vi "niScope Signalize Abort to Digitizing Process.vi"(8 "error in":errorcluster, 10 "send abort signal? (True)":bool=TRUE, 11 "niScope in":T1={"channel cfg"=[], "sessions"=[], "multi cards"=FALSE, "channels"=0, "type"=enum."n/a", "memory [B/chn]"=0, "ext. clock [Hz]"=0.0, "samples count"=0, "use streaming"=FALSE, "proc setup"={"packet size [smpl]"=0, "current timeout [s]"=0.0, "blk2blk timeout [s]"=0.0, "event time"=timestamp(0 s since 1904-01-01), "temp sampl T [s]"=0.0, "data queue"=refnum, "stop notifier"=refnum, "proc ref"=refnum}, "sample width [B]"=0, "ranges [V]"=[], "trigger setup"={"coupling"=1, "level [V]"=0.0, "slope"=0, "mode"=enum."Immediate"}, "fs [Hz]"=0.0, "bitres [bit]"=0} {"trigger setup"."level [V]" format="%.2f"; "trigger setup"."coupling" items=["AC"=0, "DC"=1, "HF Reject"=3, "LF Reject"=4, "AC Plus HF Reject"=1001]; "channel cfg"."Range [Vpk]" min=0.0; "channel cfg"."Channel" min=0}) -> (0 "error out (copy)":errorcluster, 3 "niScope out (copy)":T1={"channel cfg"=[], "sessions"=[], "multi cards"=FALSE, "channels"=0, "type"=enum."n/a", "memory [B/chn]"=0, "ext. clock [Hz]"=0.0, "samples count"=0, "use streaming"=FALSE, "proc setup"={"packet size [smpl]"=0, "current timeout [s]"=0.0, "blk2blk timeout [s]"=0.0, "event time"=timestamp(0 s since 1904-01-01), "temp sampl T [s]"=0.0, "data queue"=refnum, "stop notifier"=refnum, "proc ref"=refnum}, "sample width [B]"=0, "ranges [V]"=[], "trigger setup"={"coupling"=1, "level [V]"=0.0, "slope"=0, "mode"=enum."Immediate"}, "fs [Hz]"=0.0, "bitres [bit]"=0} {"trigger setup"."level [V]" format="%.2f"; "trigger setup"."coupling" items=["AC"=0, "DC"=1, "HF Reject"=3, "LF Reject"=4, "AC Plus HF Reject"=1001]; "channel cfg"."Range [Vpk]" min=0.0; "channel cfg"."Channel" min=0})   [LabVIEW 2018, in "niScope Virtual Digitizer.lvlib"]
doc: "This will signalize abort action to the digitizing process. This is \"gentle\" version of \"niScope Abort Digitizing on Virtual Channels\". Instead of aborting the digitizing process immediatelly by low level drivers it will just sent notification to the process and it will stop the digitizing of the cards in a controlled way. When this is called continue fetching as ussual until fetch VI returnes 'fetching done?' flag. If some data were already digitized it will be returned. The VI ignroes input error and will not generate any error."
uses:
  niScope Virtual Digitizer.lvlib
  niScope Session.ctl
  niScope Virtual Channel Config.ctl
  niScope Virtual Channel Mode.ctl
  niScope Virtual Channel Input Z.ctl
  niScope Virtual Channel Coupling.ctl
  niScope Type.ctl
  niScope Digitizing Process Options.ctl
  niScope Data Packet.ctl
  niScope Trigger Setup.ctl
  <instrlib>/niScope/Controls/niScope trigger coupling.ctl
  <instrlib>/niScope/Controls/niScope trigger slope.ctl
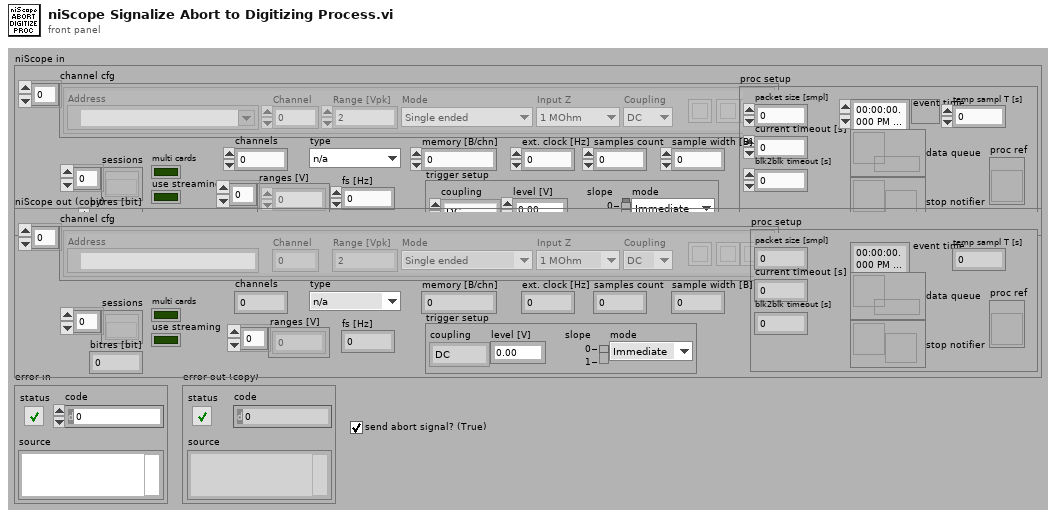
[diagram p1: front panel]
types:
  T1 = typedef "niScope Virtual Digitizer.lvlib/niScope Session.ctl" = cluster{"channel cfg":T2[], "sessions":refnum<k20>[], "multi cards":bool, "channels":i32, "type":T6, "memory [B/chn]":i32, "ext. clock [Hz]":dbl, "samples count":i64, "use streaming":bool, "proc setup":T7, "sample width [B]":i32, "ranges [V]":dbl[], "trigger setup":T8, "fs [Hz]":dbl, "bitres [bit]":i32}
  T2 = typedef "niScope Virtual Digitizer.lvlib/niScope Virtual Channel Config.ctl" = cluster{"Address":refnum<k15>, "Channel":i32, "Mode":T3, "Input Z":T4, "Coupling":T5, "Range [Vpk]":dbl, "btn clr":bool, "btn up":bool, "btn down":bool}
  T3 = typedef "niScope Virtual Digitizer.lvlib/niScope Virtual Channel Mode.ctl" = enum16{"Single ended", "Unbal. differential", "Differential"}
  T4 = typedef "niScope Virtual Digitizer.lvlib/niScope Virtual Channel Input Z.ctl" = enum16{"1 MOhm", "50 Ohm"}
  T5 = typedef "niScope Virtual Digitizer.lvlib/niScope Virtual Channel Coupling.ctl" = enum16{"AC", "DC", "GND"}
  T6 = typedef "niScope Virtual Digitizer.lvlib/niScope Type.ctl" = enum16{"n/a", "5922"}
  T7 = typedef "niScope Virtual Digitizer.lvlib/niScope Digitizing Process Options.ctl" = cluster{"packet size [smpl]":i64, "current timeout [s]":dbl, "blk2blk timeout [s]":dbl, "event time":timestamp, "temp sampl T [s]":dbl, "data queue":refnum<queue>, "stop notifier":refnum<notifier>, "proc ref":refnum<vi>}
  T8 = typedef "niScope Virtual Digitizer.lvlib/niScope Trigger Setup.ctl" = cluster{"coupling":T9, "level [V]":dbl, "slope":T10, "mode":enum16{"Immediate", "External", "Level"}}
  T9 = typedef "niScope trigger coupling.ctl" = u16
  T10 = typedef "niScope trigger slope.ctl" = i32
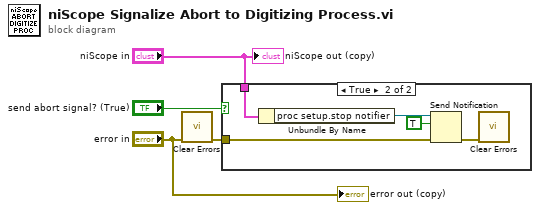
[diagram p0: block diagram]
diagram:
  n1 = call <vilib>:"Clear Errors.vi"("error in (no error)"="error in") -> ("error out"=w1:errorcluster)  [unwired: 5 in, 1 out]
  n2 = case shown="True" "send abort signal? (True)" {
    tunnel: w1 -> [_ w5]
    tunnel: "niScope in" -> [_ w6]
    frame False {
    }
    frame True {
      n3 = Unbundle By Name(w6) -> ("proc setup.stop notifier"=w9:refnum<notifier>)
      n4 = Send Notification(notification=TRUE, notifier=w9, error in (no error)=w5) -> (error out=w7:errorcluster)  [unwired: 1 out]
      n5 = call <vilib>:"Clear Errors.vi"("error in (no error)"=w7) -> ()  [unwired: 5 in, 2 out]
    }
  }
  "error out (copy)" <- "error in"
  "niScope out (copy)" <- "niScope in"
